vi "Handle Error.vi"(8 "error in (no error)":errorcluster, 11 "Mediator In":refnum<class "Mediator.lvclass">) -> (0 "error out":errorcluster, 2 "stop actor?":bool=TRUE, 3 "Mediator Out":refnum<class "Mediator.lvclass">)   [LabVIEW 2018, in "MVA Framework.lvlib" / "Mediator.lvlib" / "Mediator.lvclass"]
doc: "(<B>Filename</B>: Actor Framework.lvlib:Actor.lvclass:Handle Error.vi)\n\nDefines how the actor handles an error that occurred while processing a message. By default, this method does nothing except stop the actor."
uses:
  Mediator.lvclass
  composed-event-logger/Source/Composed Log/Types/Log Level.ctl
  composed-event-logger/Source/Composed Log/Composed Log.lvlib
  IMediator/IMediator/IMediator.lvclass
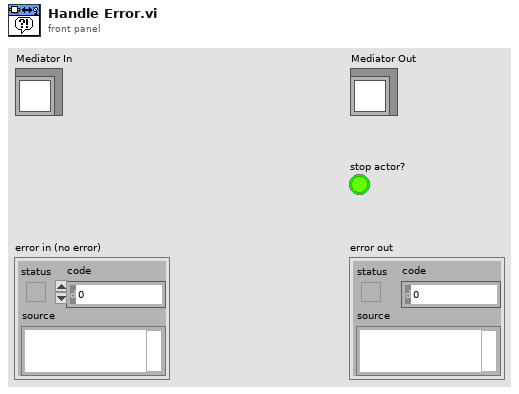
[diagram p1: front panel]
types:
  T1 = typedef "MVA Framework.lvlib/Composed Log.lvlib/Log Level.ctl" = enum16{"Debug", "Info", "Warning", "Error", "Critical"}
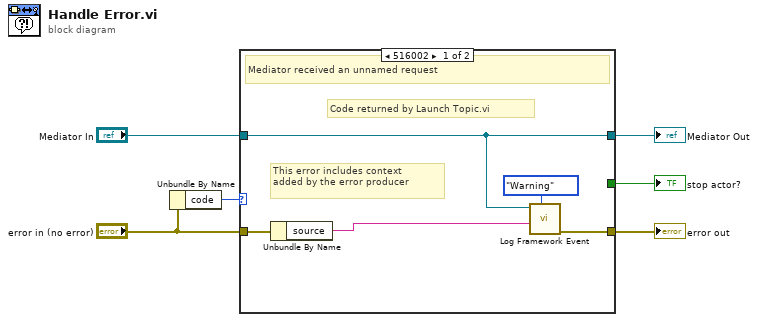
[diagram p0: block diagram]
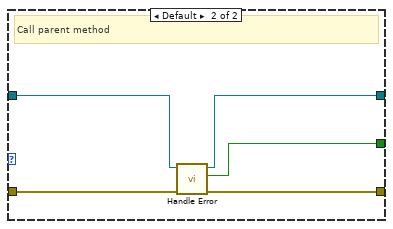
[diagram p2: hidden frame]
diagram:
  n1 = Unbundle By Name("error in (no error)") -> ("code"=w1:i32)
  n2 = case shown="516002" w1 {
    tunnel: [w9 w16] -> w6
    tunnel: [_ w15] -> w5
    tunnel: [w10 w14] -> w4
    tunnel: "error in (no error)" -> [w8 w13]
    tunnel: "Mediator In" -> [w10 w12]
    frame 516002 {
      # "Code returned by Launch Topic.vi"
      # "This error includes context\nadded by the error producer"
      # "Mediator received an unnamed request"
      n3 = Unbundle By Name(w8) -> ("source"=w7:string)
      n4 = call "Log Framework Event.vi"("Event Level (Debug)"=Log_Level."Warning", "Data To Log"=w7, "IMediator In"=w10) -> ("error out"=w9:errorcluster)  [unwired: 8 in]
    }
    frame Default {
      # "Call parent method"
      n5 = call-parent "Handle Error.vi"("error in (no error)"=w13, "IMediator In"=w12) -> ("error out"=w16:errorcluster, "stop actor?"=w15:bool, "IMediator Out"=w14:refnum<class "Mediator.lvclass">)  [unwired: 7 in]
    }
  }
  "Mediator Out" <- w4
  "error out" <- w6
  "stop actor?" <- w5
